vi "exit.vi"(8 "error in (no error)":errorcluster, 9 "Parameters":T1, 10 "Model in":refnum<class "Model.lvclass">, 11 "StandbyState in":refnum<class "StandbyState.lvclass">) -> (0 "error out":errorcluster, 2 "Model out":refnum<class "Model.lvclass">, 3 "StandbyState out":refnum<class "StandbyState.lvclass">)   [LabVIEW 2016, in "StandbyState.lvclass"]
uses:
  StandbyState.lvclass
  Model/Model.lvclass
  DataTypes/Topics/CommandExit.ctl
  DataTypes/Topics/Parts/CommandId.ctl
  DataTypes/Topics/Parts/DetailedStates.ctl
  Model/Model.lvclass/Model.ctl
  Publisher/Publisher.lvclass/Publisher.ctl
  Communicator/M1M3SAL/M1M3SAL.lvclass/M1M3SAL.ctl
  Publisher/transmit.vi
  Communicator/M1M3SAL/transmit.vi
  Communicator/M1M3SAL/write.vi
  Model/populateEventSummaryState.vi
  Model/publishEventSummaryState.vi
  Model/populateEventDetailedState.vi
  Model/publishEventDetailedState.vi
  DataTypes/Topics/M1M3SupportTopics.lvlib
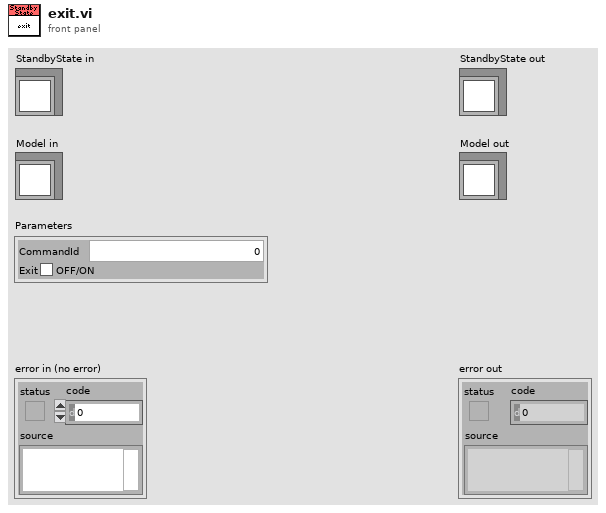
[diagram p1: front panel]
types:
  T1 = typedef "M1M3SupportTopics.lvlib/CommandExit.ctl" = cluster{"CommandId":T2, "Exit":bool}
  T2 = typedef "M1M3SupportTopics.lvlib/CommandId.ctl" = i32
  T3 = typedef "M1M3SupportTopics.lvlib/DetailedStates.ctl" = enum16{"OfflineState", "InitialState", "StandbyState", "DisabledState", "ParkedState", "FaultState", "ParkedMaintenanceState", "ActiveMaintenanceState"}
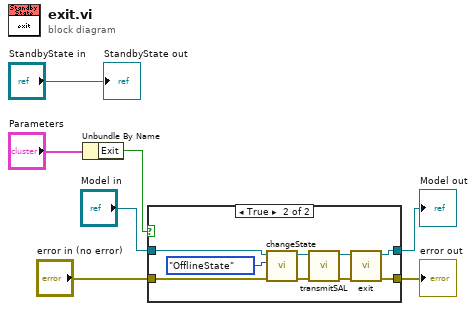
[diagram p0: block diagram]
diagram:
  n1 = Unbundle By Name("Parameters") -> ("Exit"=w6:bool)
  n2 = case shown="True" w6 {
    tunnel: "error in (no error)" -> [w8 w17]
    tunnel: [w8 w16] -> w4
    tunnel: "Model in" -> [w9 w15]
    tunnel: [w9 w14] -> w2
    frame False {
    }
    frame True {
      n3 = call "changeState.vi"("error in (no error)"=w17, "DetailedStates"=DetailedStates."OfflineState", "Model in"=w15) -> ("error out"=w10:errorcluster, "Model out"=w13:refnum<class "Model.lvclass">)  [unwired: 7 in]
      n4 = call "transmitSAL.vi"("error in (no error)"=w10, "Model in"=w13) -> ("error out"=w11:errorcluster, "Model out"=w12:refnum<class "Model.lvclass">)  [unwired: 8 in]
      n5 = call "exit.vi"("error in (no error)"=w11, "Model in"=w12) -> ("error out"=w16:errorcluster, "Model out"=w14:refnum<class "Model.lvclass">)  [unwired: 8 in]
    }
  }
  "error out" <- w4
  "Model out" <- w2
  "StandbyState out" <- "StandbyState in"
